vi "Test Asic Max P Min N Max N Min P.vi"(0 "Config Test IN":T1={"Config HW"={"VISA Rigol DP832"="Rigol_DP832", "Config Rigol DP832"=[{"Channel"=0, "V Limit"=5.5, "I Limit"=0.5, "V Out"=5.0}, {"Channel"=1, "V Limit"=5.5, "I Limit"=0.8, "V Out"=5.0}, {"Channel"=2, "V Limit"=5.5, "I Limit"=0.2, "V Out"=0.0}], "CTA Test#"="CTA013 A", "FT_Handle"=0, "Espera acceso FT"=10, "VISA Tek MDO3104"="Rigol_DP832", "VISA Key 81160A"="Rigol_DP832"}, "Config Test"=[{"Vasic"=2.8, "Global Reset"=FALSE, "Test Register?"=FALSE, "Test ADC?"=FALSE, "Test ADC"={"Repeats ADC"=100, "Max Desviation"=0.1}, "Limits ADC"={"Low"=[1.9, 1.3, 0.65, 0.0, 1.6, 1.4, 1.4, 0.9, 2.1, 0.85, 1.9], "High"=[2.1, 1.5, 0.85, 0.1, 1.4, 1.2, 1.2, 0.7, 1.9, 0.65, 1.7]}, "Test Max PN Min NP?"=FALSE, "Limits Max PN Min NP"={"Max P Upper"=2.177000045776367, "Min P Upper"=1.474, "Max N Upper"=1.475, "Min N Upper"=0.818, "Max P Lower"=1.888, "Min P Lower "=1.321, "Max N Lower"=1.322, "Min N Lower"=0.73}, "Test Rate Scan?"=FALSE, "Vin Rate Scan"=[], "Limits Rate Scan"={"High"=[0.15, 0.242, 0.331, 0.425, 0.512, 0.6, 0.688, 0.774, 0.847, 0.91], "Low"=[0.021, 0.11, 0.189, 0.27, 0.347, 0.421, 0.487, 0.551, 0.601, 0.635]}, "Test Rate Scan Adders?"=FALSE, "Vin Rate Adders"=[], "Limits Rate Scan adders"={"High"=[], "Low"=[]}, "Test offset analog?"=FALSE, "Lim Offset Analog"={"Max Analog"=0.05, "Min Analog"=-0.05}, "Test offset digital?"=FALSE, "Lim offset Dig"={"Max Dig"=0.05}, "Vasic real f.a."=2.8, "IBIAS"=FALSE, "VALUE IBIAS"=63}, {"Vasic"=2.8, "Global Reset"=FALSE, "Test Register?"=FALSE, "Test ADC?"=FALSE, "Test ADC"={"Repeats ADC"=100, "Max Desviation"=0.1}, "Limits ADC"={"Low"=[1.9, 1.3, 0.65, 0.0, 1.6, 1.4, 1.4, 0.9, 2.1, 0.85, 1.9], "High"=[2.1, 1.5, 0.85, 0.1, 1.4, 1.2, 1.2, 0.7, 1.9, 0.65, 1.7]}, "Test Max PN Min NP?"=FALSE, "Limits Max PN Min NP"={"Max P Upper"=2.177000045776367, "Min P Upper"=1.474, "Max N Upper"=1.475, "Min N Upper"=0.818, "Max P Lower"=1.888, "Min P Lower "=1.321, "Max N Lower"=1.322, "Min N Lower"=0.73}, "Test Rate Scan?"=FALSE, "Vin Rate Scan"=[], "Limits Rate Scan"={"High"=[0.15, 0.242, 0.331, 0.425, 0.512, 0.6, 0.688, 0.774, 0.847, 0.91], "Low"=[0.021, 0.11, 0.189, 0.27, 0.347, 0.421, 0.487, 0.551, 0.601, 0.635]}, "Test Rate Scan Adders?"=FALSE, "Vin Rate Adders"=[], "Limits Rate Scan adders"={"High"=[], "Low"=[]}, "Test offset analog?"=FALSE, "Lim Offset Analog"={"Max Analog"=0.05, "Min Analog"=-0.05}, "Test offset digital?"=FALSE, "Lim offset Dig"={"Max Dig"=0.05}, "Vasic real f.a."=2.8, "IBIAS"=FALSE, "VALUE IBIAS"=63}, {"Vasic"=2.8, "Global Reset"=FALSE, "Test Register?"=FALSE, "Test ADC?"=FALSE, "Test ADC"={"Repeats ADC"=100, "Max Desviation"=0.1}, "Limits ADC"={"Low"=[1.9, 1.3, 0.65, 0.0, 1.6, 1.4, 1.4, 0.9, 2.1, 0.85, 1.9], "High"=[2.1, 1.5, 0.85, 0.1, 1.4, 1.2, 1.2, 0.7, 1.9, 0.65, 1.7]}, "Test Max PN Min NP?"=FALSE, "Limits Max PN Min NP"={"Max P Upper"=2.177000045776367, "Min P Upper"=1.474, "Max N Upper"=1.475, "Min N Upper"=0.818, "Max P Lower"=1.888, "Min P Lower "=1.321, "Max N Lower"=1.322, "Min N Lower"=0.73}, "Test Rate Scan?"=FALSE, "Vin Rate Scan"=[], "Limits Rate Scan"={"High"=[0.15, 0.242, 0.331, 0.425, 0.512, 0.6, 0.688, 0.774, 0.847, 0.91], "Low"=[0.021, 0.11, 0.189, 0.27, 0.347, 0.421, 0.487, 0.551, 0.601, 0.635]}, "Test Rate Scan Adders?"=FALSE, "Vin Rate Adders"=[], "Limits Rate Scan adders"={"High"=[], "Low"=[]}, "Test offset analog?"=FALSE, "Lim Offset Analog"={"Max Analog"=0.05, "Min Analog"=-0.05}, "Test offset digital?"=FALSE, "Lim offset Dig"={"Max Dig"=0.05}, "Vasic real f.a."=2.8, "IBIAS"=FALSE, "VALUE IBIAS"=63}, {"Vasic"=2.8, "Global Reset"=FALSE, "Test Register?"=FALSE, "Test ADC?"=FALSE, "Test ADC"={"Repeats ADC"=100, "Max Desviation"=0.1}, "Limits ADC"={"Low"=[1.9, 1.3, 0.65, 0.0, 1.6, 1.4, 1.4, 0.9, 2.1, 0.85, 1.9], "High"=[2.1, 1.5, 0.85, 0.1, 1.4, 1.2, 1.2, 0.7, 1.9, 0.65, 1.7]}, "Test Max PN Min NP?"=FALSE, "Limits Max PN Min NP"={"Max P Upper"=2.177000045776367, "Min P Upper"=1.474, "Max N Upper"=1.475, "Min N Upper"=0.818, "Max P Lower"=1.888, "Min P Lower "=1.321, "Max N Lower"=1.322, "Min N Lower"=0.73}, "Test Rate Scan?"=FALSE, "Vin Rate Scan"=[], "Limits Rate Scan"={"High"=[0.15, 0.242, 0.331, 0.425, 0.512, 0.6, 0.688, 0.774, 0.847, 0.91], "Low"=[0.021, 0.11, 0.189, 0.27, 0.347, 0.421, 0.487, 0.551, 0.601, 0.635]}, "Test Rate Scan Adders?"=FALSE, "Vin Rate Adders"=[], "Limits Rate Scan adders"={"High"=[], "Low"=[]}, "Test offset analog?"=FALSE, "Lim Offset Analog"={"Max Analog"=0.05, "Min Analog"=-0.05}, "Test offset digital?"=FALSE, "Lim offset Dig"={"Max Dig"=0.05}, "Vasic real f.a."=2.8, "IBIAS"=FALSE, "VALUE IBIAS"=63}], "Result"=[], "Execucion Test"={"Vasic Actual"=0}, "Config VGA"={"Theoretical Voltage"=[], "Real Voltage"=[102.85, 207.14, 299.57, 404.85, 495.71, 606.85, 697.71, 801.14, 897.14, 998.85], "Pulse Width"=57344, "Frecuency Pulse"=1000000.0, "VGA Gain"=[9, 16, 24, 34, 43, 52, 61, 72, 81, 93]}, "Test Info"={"Asic"="", "Operator"="", "Place"="", "Time start"=timestamp(0 s since 1904-01-01), "Time stop"=timestamp(0 s since 1904-01-01)}, "Info machine"={"SO"="", "SO Name"="", "SO Ver"="", "SO Build"="", "CPU"="", "APP"="", "APP YEAR"="", "APP ver"="", "APP User"="", "APP Serail"="", "MAC"=[], "PC NAME"=[], "PC IP"=[], "BIOS MANU"="", "BIOS NAME"="", "BIOS SERIAL"="", "BOARD MANU"="", "BOARD NAME"="", "BOARD SERIAL"="", "Driver Version"="", "Library Version"="", "FPGA Ver"=0, "ID CTA board"=0, "LAST BOOT"="", "LABVIEW Ver"=0}, "Partial Report"="", "CONFIG GEN"=[]} {"CONFIG GEN"."Vasic Theorical" min=1.0 max=1000000.0 step=1.0 format="%#_6pV"; "CONFIG GEN"."Frequency" min=0.001 max=333000000.0 step=1000.0 format="%#_6pHz"; "CONFIG GEN"."Leading Edge Time" min=1e-09 max=1.0 step=1e-10 format="%#_6ps"; "CONFIG GEN"."Trailing Edge Time" min=1e-09 max=1.0 step=1e-10 format="%#_6ps"; "CONFIG GEN"."Delay" min=0.0 max=1.0 step=1e-12 format="%#_6ps"; "CONFIG GEN"."Trigger Level Sync" items=["ECL", "TTL"]; "CONFIG GEN"."Trigger Sync Out" items=["AB"=3, "B"=2, "A"=1, "None"=0]; "CONFIG GEN"."Load" min=1.0 max=1000000.0 step=1.0 format="%#_6p"; "CONFIG GEN"."DC Offset" min=-10.0 max=10.0 step=0.1 format="%#_6pV"; "CONFIG GEN"."Amplitude" min=0.05 max=5.0 step=0.001 format="%#_6pV"; "CONFIG GEN"."Width Time" min=1.5e-09 max=1.0 step=1e-10 format="%#_6ps"; "CONFIG GEN"."Channel" items=["Channel1"=1, "Channel2"=2]; "Config VGA"."Theoretical Voltage" format="%1.4f"; "Config VGA"."VGA Gain" format="%02x"; "Config VGA"."Frecuency Pulse" format="%0_2p"; "Config VGA"."Pulse Width" format="%04x"; "Config VGA"."Real Voltage" format="%1.5f"; "Config Test"."VALUE IBIAS" max=63 step=1; "Config Test"."Vasic real f.a." min=2.8 max=3.8 step=0.01 format="%.2g"; "Config Test"."Limits Rate Scan adders"."Low" format="%1.3f"; "Config Test"."Limits Rate Scan adders"."High" format="%1.3f"; "Config Test"."Limits ADC"."High" format="%1.4f"; "Config Test"."Limits ADC"."Low" format="%1.3f"; "Config Test"."Lim offset Dig"."Max Dig" format="%.3g"; "Config Test"."Lim Offset Analog"."Min Analog" format="%.3g"; "Config Test"."Lim Offset Analog"."Max Analog" format="%.3g"; "Config Test"."Limits Rate Scan"."Low" format="%1.4f"; "Config Test"."Limits Rate Scan"."High" format="%1.3f"; "Config Test"."Limits Max PN Min NP"."Min P Upper" format="%.3g"; "Config Test"."Limits Max PN Min NP"."Min P Lower" format="%.3g"; "Config Test"."Limits Max PN Min NP"."Max N Lower" format="%.3g"; "Config Test"."Limits Max PN Min NP"."Max N Upper" format="%.3g"; "Config Test"."Limits Max PN Min NP"."Min N Lower" format="%.3g"; "Config Test"."Limits Max PN Min NP"."Min N Upper" format="%.3g"; "Config Test"."Limits Max PN Min NP"."Max P Upper" format="%.3g"; "Config Test"."Limits Max PN Min NP"."Max P Lower" format="%.3g"; "Config Test"."Vasic" min=2.8 max=3.8 step=0.01 format="%.2g"; "Config HW"."Config Rigol DP832"."Channel" items=["+30V Channel 1", "+30V Channel 2", "+5V Channel 3"]; "Config HW"."Config Rigol DP832"."V Limit" format="%.1g"; "Config HW"."Config Rigol DP832"."I Limit" format="%.1g"; "Config HW"."Config Rigol DP832"."V Out" format="%.1g"; "Result"."Test Registros"."Read W/R" format="%04x"; "Result"."Test Registros"."Pattern W/R" format="%04x"; "Result"."Test Registros"."Read Default" format="%04x"; "Result"."Test Registros"."Pattern Default" format="%04x"}, 11 "Error IN":errorcluster) -> (4 "Config Test OUT":T1={"Config HW"={"VISA Rigol DP832"="Rigol_DP832", "Config Rigol DP832"=[{"Channel"=0, "V Limit"=5.5, "I Limit"=0.5, "V Out"=5.0}, {"Channel"=1, "V Limit"=5.5, "I Limit"=0.8, "V Out"=5.0}, {"Channel"=2, "V Limit"=5.5, "I Limit"=0.2, "V Out"=0.0}], "CTA Test#"="CTA013 A", "FT_Handle"=0, "Espera acceso FT"=10, "VISA Tek MDO3104"="Rigol_DP832", "VISA Key 81160A"="Rigol_DP832"}, "Config Test"=[{"Vasic"=2.8, "Global Reset"=FALSE, "Test Register?"=FALSE, "Test ADC?"=FALSE, "Test ADC"={"Repeats ADC"=100, "Max Desviation"=0.1}, "Limits ADC"={"Low"=[1.9, 1.3, 0.65, 0.0, 1.6, 1.4, 1.4, 0.9, 2.1, 0.85, 1.9], "High"=[2.1, 1.5, 0.85, 0.1, 1.4, 1.2, 1.2, 0.7, 1.9, 0.65, 1.7]}, "Test Max PN Min NP?"=FALSE, "Limits Max PN Min NP"={"Max P Upper"=2.177000045776367, "Min P Upper"=1.474, "Max N Upper"=1.475, "Min N Upper"=0.818, "Max P Lower"=1.888, "Min P Lower "=1.321, "Max N Lower"=1.322, "Min N Lower"=0.73}, "Test Rate Scan?"=FALSE, "Vin Rate Scan"=[], "Limits Rate Scan"={"High"=[0.15, 0.242, 0.331, 0.425, 0.512, 0.6, 0.688, 0.774, 0.847, 0.91], "Low"=[0.021, 0.11, 0.189, 0.27, 0.347, 0.421, 0.487, 0.551, 0.601, 0.635]}, "Test Rate Scan Adders?"=FALSE, "Vin Rate Adders"=[], "Limits Rate Scan adders"={"High"=[], "Low"=[]}, "Test offset analog?"=FALSE, "Lim Offset Analog"={"Max Analog"=0.05, "Min Analog"=-0.05}, "Test offset digital?"=FALSE, "Lim offset Dig"={"Max Dig"=0.05}, "Vasic real f.a."=2.8, "IBIAS"=FALSE, "VALUE IBIAS"=63}, {"Vasic"=2.8, "Global Reset"=FALSE, "Test Register?"=FALSE, "Test ADC?"=FALSE, "Test ADC"={"Repeats ADC"=100, "Max Desviation"=0.1}, "Limits ADC"={"Low"=[1.9, 1.3, 0.65, 0.0, 1.6, 1.4, 1.4, 0.9, 2.1, 0.85, 1.9], "High"=[2.1, 1.5, 0.85, 0.1, 1.4, 1.2, 1.2, 0.7, 1.9, 0.65, 1.7]}, "Test Max PN Min NP?"=FALSE, "Limits Max PN Min NP"={"Max P Upper"=2.177000045776367, "Min P Upper"=1.474, "Max N Upper"=1.475, "Min N Upper"=0.818, "Max P Lower"=1.888, "Min P Lower "=1.321, "Max N Lower"=1.322, "Min N Lower"=0.73}, "Test Rate Scan?"=FALSE, "Vin Rate Scan"=[], "Limits Rate Scan"={"High"=[0.15, 0.242, 0.331, 0.425, 0.512, 0.6, 0.688, 0.774, 0.847, 0.91], "Low"=[0.021, 0.11, 0.189, 0.27, 0.347, 0.421, 0.487, 0.551, 0.601, 0.635]}, "Test Rate Scan Adders?"=FALSE, "Vin Rate Adders"=[], "Limits Rate Scan adders"={"High"=[], "Low"=[]}, "Test offset analog?"=FALSE, "Lim Offset Analog"={"Max Analog"=0.05, "Min Analog"=-0.05}, "Test offset digital?"=FALSE, "Lim offset Dig"={"Max Dig"=0.05}, "Vasic real f.a."=2.8, "IBIAS"=FALSE, "VALUE IBIAS"=63}, {"Vasic"=2.8, "Global Reset"=FALSE, "Test Register?"=FALSE, "Test ADC?"=FALSE, "Test ADC"={"Repeats ADC"=100, "Max Desviation"=0.1}, "Limits ADC"={"Low"=[1.9, 1.3, 0.65, 0.0, 1.6, 1.4, 1.4, 0.9, 2.1, 0.85, 1.9], "High"=[2.1, 1.5, 0.85, 0.1, 1.4, 1.2, 1.2, 0.7, 1.9, 0.65, 1.7]}, "Test Max PN Min NP?"=FALSE, "Limits Max PN Min NP"={"Max P Upper"=2.177000045776367, "Min P Upper"=1.474, "Max N Upper"=1.475, "Min N Upper"=0.818, "Max P Lower"=1.888, "Min P Lower "=1.321, "Max N Lower"=1.322, "Min N Lower"=0.73}, "Test Rate Scan?"=FALSE, "Vin Rate Scan"=[], "Limits Rate Scan"={"High"=[0.15, 0.242, 0.331, 0.425, 0.512, 0.6, 0.688, 0.774, 0.847, 0.91], "Low"=[0.021, 0.11, 0.189, 0.27, 0.347, 0.421, 0.487, 0.551, 0.601, 0.635]}, "Test Rate Scan Adders?"=FALSE, "Vin Rate Adders"=[], "Limits Rate Scan adders"={"High"=[], "Low"=[]}, "Test offset analog?"=FALSE, "Lim Offset Analog"={"Max Analog"=0.05, "Min Analog"=-0.05}, "Test offset digital?"=FALSE, "Lim offset Dig"={"Max Dig"=0.05}, "Vasic real f.a."=2.8, "IBIAS"=FALSE, "VALUE IBIAS"=63}, {"Vasic"=2.8, "Global Reset"=FALSE, "Test Register?"=FALSE, "Test ADC?"=FALSE, "Test ADC"={"Repeats ADC"=100, "Max Desviation"=0.1}, "Limits ADC"={"Low"=[1.9, 1.3, 0.65, 0.0, 1.6, 1.4, 1.4, 0.9, 2.1, 0.85, 1.9], "High"=[2.1, 1.5, 0.85, 0.1, 1.4, 1.2, 1.2, 0.7, 1.9, 0.65, 1.7]}, "Test Max PN Min NP?"=FALSE, "Limits Max PN Min NP"={"Max P Upper"=2.177000045776367, "Min P Upper"=1.474, "Max N Upper"=1.475, "Min N Upper"=0.818, "Max P Lower"=1.888, "Min P Lower "=1.321, "Max N Lower"=1.322, "Min N Lower"=0.73}, "Test Rate Scan?"=FALSE, "Vin Rate Scan"=[], "Limits Rate Scan"={"High"=[0.15, 0.242, 0.331, 0.425, 0.512, 0.6, 0.688, 0.774, 0.847, 0.91], "Low"=[0.021, 0.11, 0.189, 0.27, 0.347, 0.421, 0.487, 0.551, 0.601, 0.635]}, "Test Rate Scan Adders?"=FALSE, "Vin Rate Adders"=[], "Limits Rate Scan adders"={"High"=[], "Low"=[]}, "Test offset analog?"=FALSE, "Lim Offset Analog"={"Max Analog"=0.05, "Min Analog"=-0.05}, "Test offset digital?"=FALSE, "Lim offset Dig"={"Max Dig"=0.05}, "Vasic real f.a."=2.8, "IBIAS"=FALSE, "VALUE IBIAS"=63}], "Result"=[], "Execucion Test"={"Vasic Actual"=0}, "Config VGA"={"Theoretical Voltage"=[], "Real Voltage"=[102.85, 207.14, 299.57, 404.85, 495.71, 606.85, 697.71, 801.14, 897.14, 998.85], "Pulse Width"=57344, "Frecuency Pulse"=1000000.0, "VGA Gain"=[9, 16, 24, 34, 43, 52, 61, 72, 81, 93]}, "Test Info"={"Asic"="", "Operator"="", "Place"="", "Time start"=timestamp(0 s since 1904-01-01), "Time stop"=timestamp(0 s since 1904-01-01)}, "Info machine"={"SO"="", "SO Name"="", "SO Ver"="", "SO Build"="", "CPU"="", "APP"="", "APP YEAR"="", "APP ver"="", "APP User"="", "APP Serail"="", "MAC"=[], "PC NAME"=[], "PC IP"=[], "BIOS MANU"="", "BIOS NAME"="", "BIOS SERIAL"="", "BOARD MANU"="", "BOARD NAME"="", "BOARD SERIAL"="", "Driver Version"="", "Library Version"="", "FPGA Ver"=0, "ID CTA board"=0, "LAST BOOT"="", "LABVIEW Ver"=0}, "Partial Report"="", "CONFIG GEN"=[]} {"CONFIG GEN"."Vasic Theorical" min=1.0 max=1000000.0 step=1.0 format="%#_6pV"; "CONFIG GEN"."Frequency" min=0.001 max=333000000.0 step=1000.0 format="%#_6pHz"; "CONFIG GEN"."Leading Edge Time" min=1e-09 max=1.0 step=1e-10 format="%#_6ps"; "CONFIG GEN"."Trailing Edge Time" min=1e-09 max=1.0 step=1e-10 format="%#_6ps"; "CONFIG GEN"."Delay" min=0.0 max=1.0 step=1e-12 format="%#_6ps"; "CONFIG GEN"."Trigger Level Sync" items=["ECL", "TTL"]; "CONFIG GEN"."Trigger Sync Out" items=["AB"=3, "B"=2, "A"=1, "None"=0]; "CONFIG GEN"."Load" min=1.0 max=1000000.0 step=1.0 format="%#_6p"; "CONFIG GEN"."DC Offset" min=-10.0 max=10.0 step=0.1 format="%#_6pV"; "CONFIG GEN"."Amplitude" min=0.05 max=5.0 step=0.001 format="%#_6pV"; "CONFIG GEN"."Width Time" min=1.5e-09 max=1.0 step=1e-10 format="%#_6ps"; "CONFIG GEN"."Channel" items=["Channel1"=1, "Channel2"=2]; "Config VGA"."Theoretical Voltage" format="%1.4f"; "Config VGA"."VGA Gain" format="%02x"; "Config VGA"."Frecuency Pulse" format="%0_2p"; "Config VGA"."Pulse Width" format="%04x"; "Config VGA"."Real Voltage" format="%1.5f"; "Config Test"."VALUE IBIAS" max=63 step=1; "Config Test"."Vasic real f.a." min=2.8 max=3.8 step=0.01 format="%.2g"; "Config Test"."Limits Rate Scan adders"."Low" format="%1.3f"; "Config Test"."Limits Rate Scan adders"."High" format="%1.3f"; "Config Test"."Limits ADC"."High" format="%1.4f"; "Config Test"."Limits ADC"."Low" format="%1.3f"; "Config Test"."Lim offset Dig"."Max Dig" format="%.3g"; "Config Test"."Lim Offset Analog"."Min Analog" format="%.3g"; "Config Test"."Lim Offset Analog"."Max Analog" format="%.3g"; "Config Test"."Limits Rate Scan"."Low" format="%1.4f"; "Config Test"."Limits Rate Scan"."High" format="%1.3f"; "Config Test"."Limits Max PN Min NP"."Min P Upper" format="%.3g"; "Config Test"."Limits Max PN Min NP"."Min P Lower" format="%.3g"; "Config Test"."Limits Max PN Min NP"."Max N Lower" format="%.3g"; "Config Test"."Limits Max PN Min NP"."Max N Upper" format="%.3g"; "Config Test"."Limits Max PN Min NP"."Min N Lower" format="%.3g"; "Config Test"."Limits Max PN Min NP"."Min N Upper" format="%.3g"; "Config Test"."Limits Max PN Min NP"."Max P Upper" format="%.3g"; "Config Test"."Limits Max PN Min NP"."Max P Lower" format="%.3g"; "Config Test"."Vasic" min=2.8 max=3.8 step=0.01 format="%.2g"; "Config HW"."Config Rigol DP832"."Channel" items=["+30V Channel 1", "+30V Channel 2", "+5V Channel 3"]; "Config HW"."Config Rigol DP832"."V Limit" format="%.1g"; "Config HW"."Config Rigol DP832"."I Limit" format="%.1g"; "Config HW"."Config Rigol DP832"."V Out" format="%.1g"; "Result"."Test Registros"."Read W/R" format="%04x"; "Result"."Test Registros"."Pattern W/R" format="%04x"; "Result"."Test Registros"."Read Default" format="%04x"; "Result"."Test Registros"."Pattern Default" format="%04x"}, 8 "Max P Min N":bool, 10 "Min P Max N":bool, 15 "Error OUT":errorcluster)   [LabVIEW 2019]
uses:
  Test.ctl
  TEST.TEST CONFIG HW.ctl
  Rigol DP832/DP832_Control Channels.ctl
  TEST.TEST CONFIG TEST MATRIZ.ctl
  TEST.TEST CONFIG TEST.ctl
  TEST.TEST RESULT.ctl
  test_result fvasic.ctl
  TEST.TEST EXECUTION TEST.ctl
  TEST.TEST CONFIG VGA.ctl
  TEST.TEST TEST INFO.ctl
  TEST.TEST INFO PC.ctl
  GenPulse_configurar.ctl
  Global.Salir Ya.vi
panel:
  in  "Tab Control":enum32{"Page 1", "Page 2"}(tab)
  out "Progress %":u8 format="%02d%%"
  out "Progress barr":u8(slide) scale=0.0..100.0
  # "Test Max P Min N / Min P Max N"
  # "Modo 2\nModo 3\nModo 4\nModo 2\nModo 3\nModo 4"
  # "Modo 2\nModo 3\nModo 4\nModo 2\nModo 3\nModo 4"
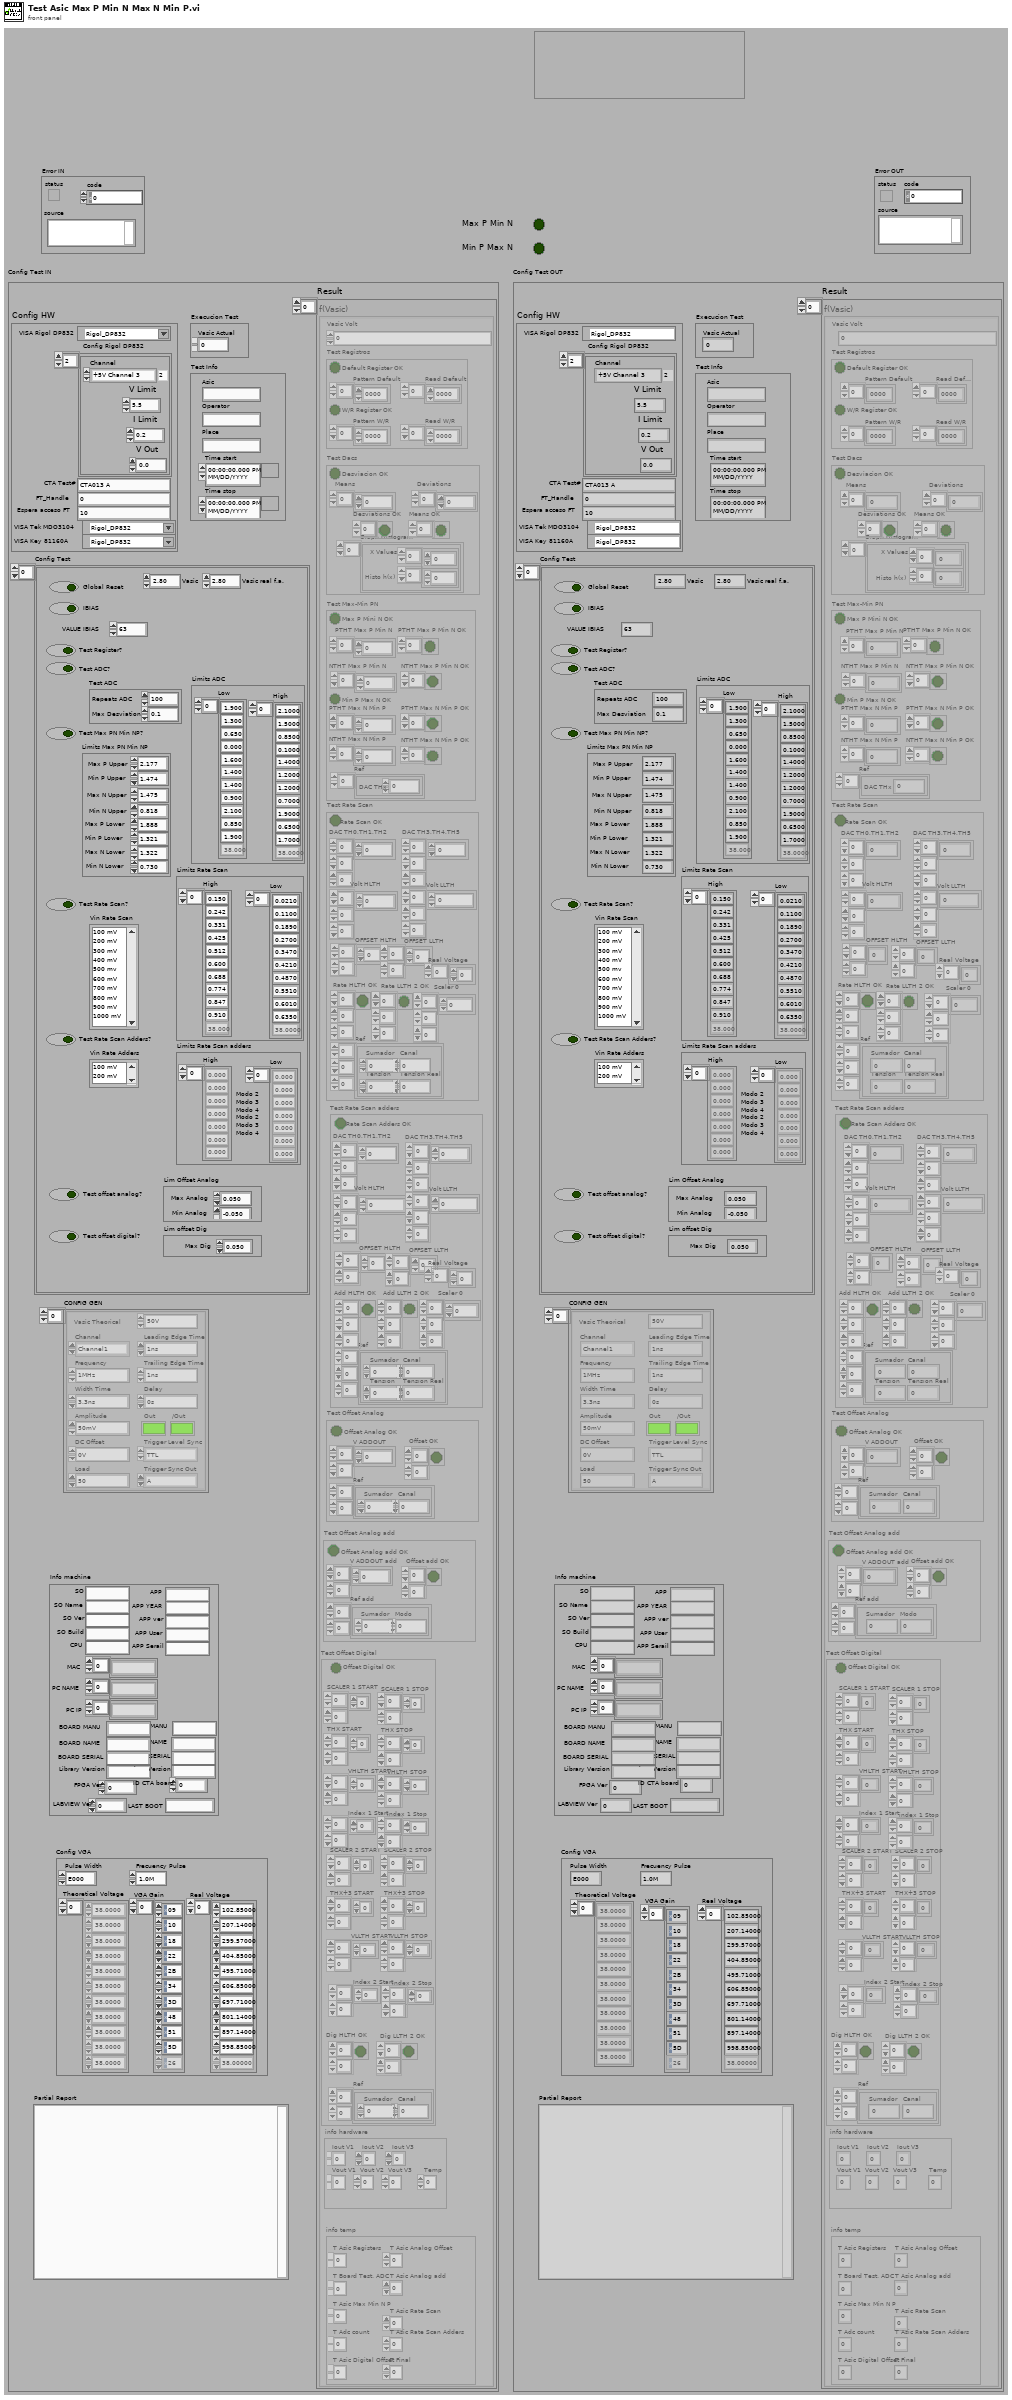
[diagram p1: front panel]
types:
  T1 = typedef "Test.ctl" = cluster{"Config HW":T2, "Config Test":T4, "Result":T6, "Execucion Test":T8, "Config VGA":T9, "Test Info":T10, "Info machine":T11, "Partial Report":string, "CONFIG GEN":T12[]}
  T2 = typedef "TEST.TEST CONFIG HW.ctl" = cluster{"VISA Rigol DP832":refnum<visa-resource-name>, "Config Rigol DP832":cluster{"Channel":T3, "V Limit":dbl, "I Limit":dbl, "V Out":dbl}[], "CTA Test#":string, "FT_Handle":u32, "Espera acceso FT":u32, "VISA Tek MDO3104":refnum<visa-resource-name>, "VISA Key 81160A":refnum<visa-resource-name>}
  T3 = typedef "DP832_Control Channels.ctl" = i32
  T4 = typedef "TEST.TEST CONFIG TEST MATRIZ.ctl" = T5[]
  T5 = typedef "TEST.TEST CONFIG TEST.ctl" = cluster{"Vasic":dbl, "Global Reset":bool, "Test Register?":bool, "Test ADC?":bool, "Test ADC":cluster{"Repeats ADC":i32, "Max Desviation":dbl}, "Limits ADC":cluster{"Low":dbl[], "High":dbl[]}, "Test Max PN Min NP?":bool, "Limits Max PN Min NP":cluster{"Max P Upper":dbl, "Min P Upper":dbl, "Max N Upper":dbl, "Min N Upper":dbl, "Max P Lower":dbl, "Min P Lower ":dbl, "Max N Lower":dbl, "Min N Lower":dbl}, "Test Rate Scan?":bool, "Vin Rate Scan":i32[], "Limits Rate Scan":cluster{"High":dbl[], "Low":dbl[]}, "Test Rate Scan Adders?":bool, "Vin Rate Adders":i32[], "Limits Rate Scan adders":cluster{"High":dbl[], "Low":dbl[]}, "Test offset analog?":bool, "Lim Offset Analog":cluster{"Max Analog":dbl, "Min Analog":dbl}, "Test offset digital?":bool, "Lim offset Dig":cluster{"Max Dig":dbl}, "Vasic real f.a.":dbl, "IBIAS":bool, "VALUE IBIAS":u8}
  T6 = typedef "TEST.TEST RESULT.ctl" = T7[]
  T7 = typedef "test_result fvasic.ctl" = cluster{"Vasic Volt":i32, "Test Registros":cluster{"Default Register OK":bool, "Pattern Default":u16[], "Read Default":u16[], "W/R Register OK":bool, "Pattern W/R":u16[], "Read W/R":u16[]}, "Test Dacs":cluster{"Desviacion OK":bool, "Means":dbl[], "Deviations":dbl[], "Desviations OK":bool[], "Means OK":bool[], "Graph Histogram":cluster{"X Values":dbl[], "Histo h(x)":i32[]}[]}, "Test Max-Min PN":cluster{"Max P Mini N OK":bool, "PTHT Max P Min N":dbl[], "PTHT Max P Min N OK":bool[], "NTHT Max P Min N":dbl[], "NTHT Max P Min N OK":bool[], "Min P Max N OK":bool, "PTHT Max N Min P":dbl[], "PTHT Max N Min P OK":bool[], "NTHT Max N Min P":dbl[], "NTHT Max N Min P OK":bool[], "Ref":cluster{"DAC THx":u8}[]}, "Test Rate Scan":cluster{"Rate Scan OK":bool, "DAC TH0,TH1,TH2":u16[][][], "Volt HLTH":dbl[][][], "Rate HLTH OK":bool[][][], "DAC TH3,TH4,TH5":u16[][][], "Volt LLTH":dbl[][][], "Rate LLTH 2 OK":bool[][][], "Scaler 0":u16[][][], "Ref":cluster{"Sumador":u8, "Canal":u8, "Tension":u8, "Tension Real":dbl}[][][], "OFFSET HLTH":dbl[][], "OFFSET LLTH":dbl[][], "Real Voltage":dbl[]}, "Test Rate Scan adders":cluster{"Rate Scan Adders OK":bool, "DAC TH0,TH1,TH2":u16[][][], "Volt HLTH":dbl[][][], "Add HLTH OK":bool[][][], "DAC TH3,TH4,TH5":u16[][][], "Volt LLTH":dbl[][][], "Add LLTH 2 OK":bool[][][], "Scaler 0":u16[][][], "Ref":cluster{"Sumador":u8, "Canal":u8, "Tension":u8, "Tension Real":dbl}[][][], "OFFSET HLTH":dbl[][], "OFFSET LLTH":dbl[][], "Real Voltage":dbl[]}, "Test Offset Analog":cluster{"Offset Analog OK":bool, "V ADDOUT":dbl[][], "Offset OK":bool[][], "Ref":cluster{"Sumador":u8, "Canal":u8}[][]}, "Test Offset Digital":cluster{"Offset Digital OK":bool, "SCALER 1 START":u16[][], "SCALER 1 STOP":u16[][], "THX START":u16[][], "THX STOP":u16[][], "VHLTH START":dbl[][], "VHLTH STOP":dbl[][], "Index 1 Start":i32[][], "index 1 Stop":i32[][], "SCALER 2 START":u16[][], "SCALER 2 STOP":u16[][], "THX+3 START":u16[][], "THX+3 STOP":u16[][], "VLLTH START":dbl[][], "VLLTH STOP":dbl[][], "Index 2 Start":i32[][], "index 2 Stop":i32[][], "Dig HLTH OK":bool[][], "Dig LLTH 2 OK":bool[][], "Ref":cluster{"Sumador":u8, "Canal":u8}[][]}, "info hardware":cluster{"Iout V1":dbl, "Iout V2":dbl, "Iout V3":dbl, "Vout V1":dbl, "Vout V2":dbl, "Vout V3":dbl, "Temp":dbl}, "Test Offset Analog add":cluster{"Offset Analog add OK":bool, "V ADDOUT add":dbl[][], "Offset add OK":bool[][], "Ref add":cluster{"Sumador":u8, "Modo":u8}[][]}, "info temp":cluster{"T Asic Registers":dbl, "T Board Test. ADC":dbl, "T Asic Max Min N P":dbl, "T Adc count":dbl, "T Asic Digital Offset":dbl, "T Asic Analog Offset":dbl, "T Asic Analog add":dbl, "T Asic Rate Scan":dbl, "T Asic Rate Scan Adders":dbl, "T Final":dbl}}
  T8 = typedef "TEST.TEST EXECUTION TEST.ctl" = cluster{"Vasic Actual":i32}
  T9 = typedef "TEST.TEST CONFIG VGA.ctl" = cluster{"Theoretical Voltage":dbl[], "Real Voltage":dbl[], "Pulse Width":u16, "Frecuency Pulse":dbl, "VGA Gain":u8[]}
  T10 = typedef "TEST.TEST TEST INFO.ctl" = cluster{"Asic":string, "Operator":string, "Place":string, "Time start":timestamp, "Time stop":timestamp}
  T11 = typedef "TEST.TEST INFO PC.ctl" = cluster{"SO":string, "SO Name":string, "SO Ver":string, "SO Build":string, "CPU":string, "APP":string, "APP YEAR":string, "APP ver":string, "APP User":string, "APP Serail":string, "MAC":string[], "PC NAME":string[], "PC IP":string[], "BIOS MANU":string, "BIOS NAME":string, "BIOS SERIAL":string, "BOARD MANU":string, "BOARD NAME":string, "BOARD SERIAL":string, "Driver Version":string, "Library Version":string, "FPGA Ver":u8, "ID CTA board":u64, "LAST BOOT":string, "LABVIEW Ver":u32}
  T12 = typedef "GenPulse_configurar.ctl" = cluster{"Channel":u16, "Frequency":dbl, "Width Time":dbl, "Amplitude":dbl, "DC Offset":dbl, "Load":dbl, "Leading Edge Time":dbl, "Trailing Edge Time":dbl, "Delay":dbl, "Out":bool, "/Out":bool, "Trigger Level Sync":u16, "Trigger Sync Out":u16, "Vasic Theorical":dbl}
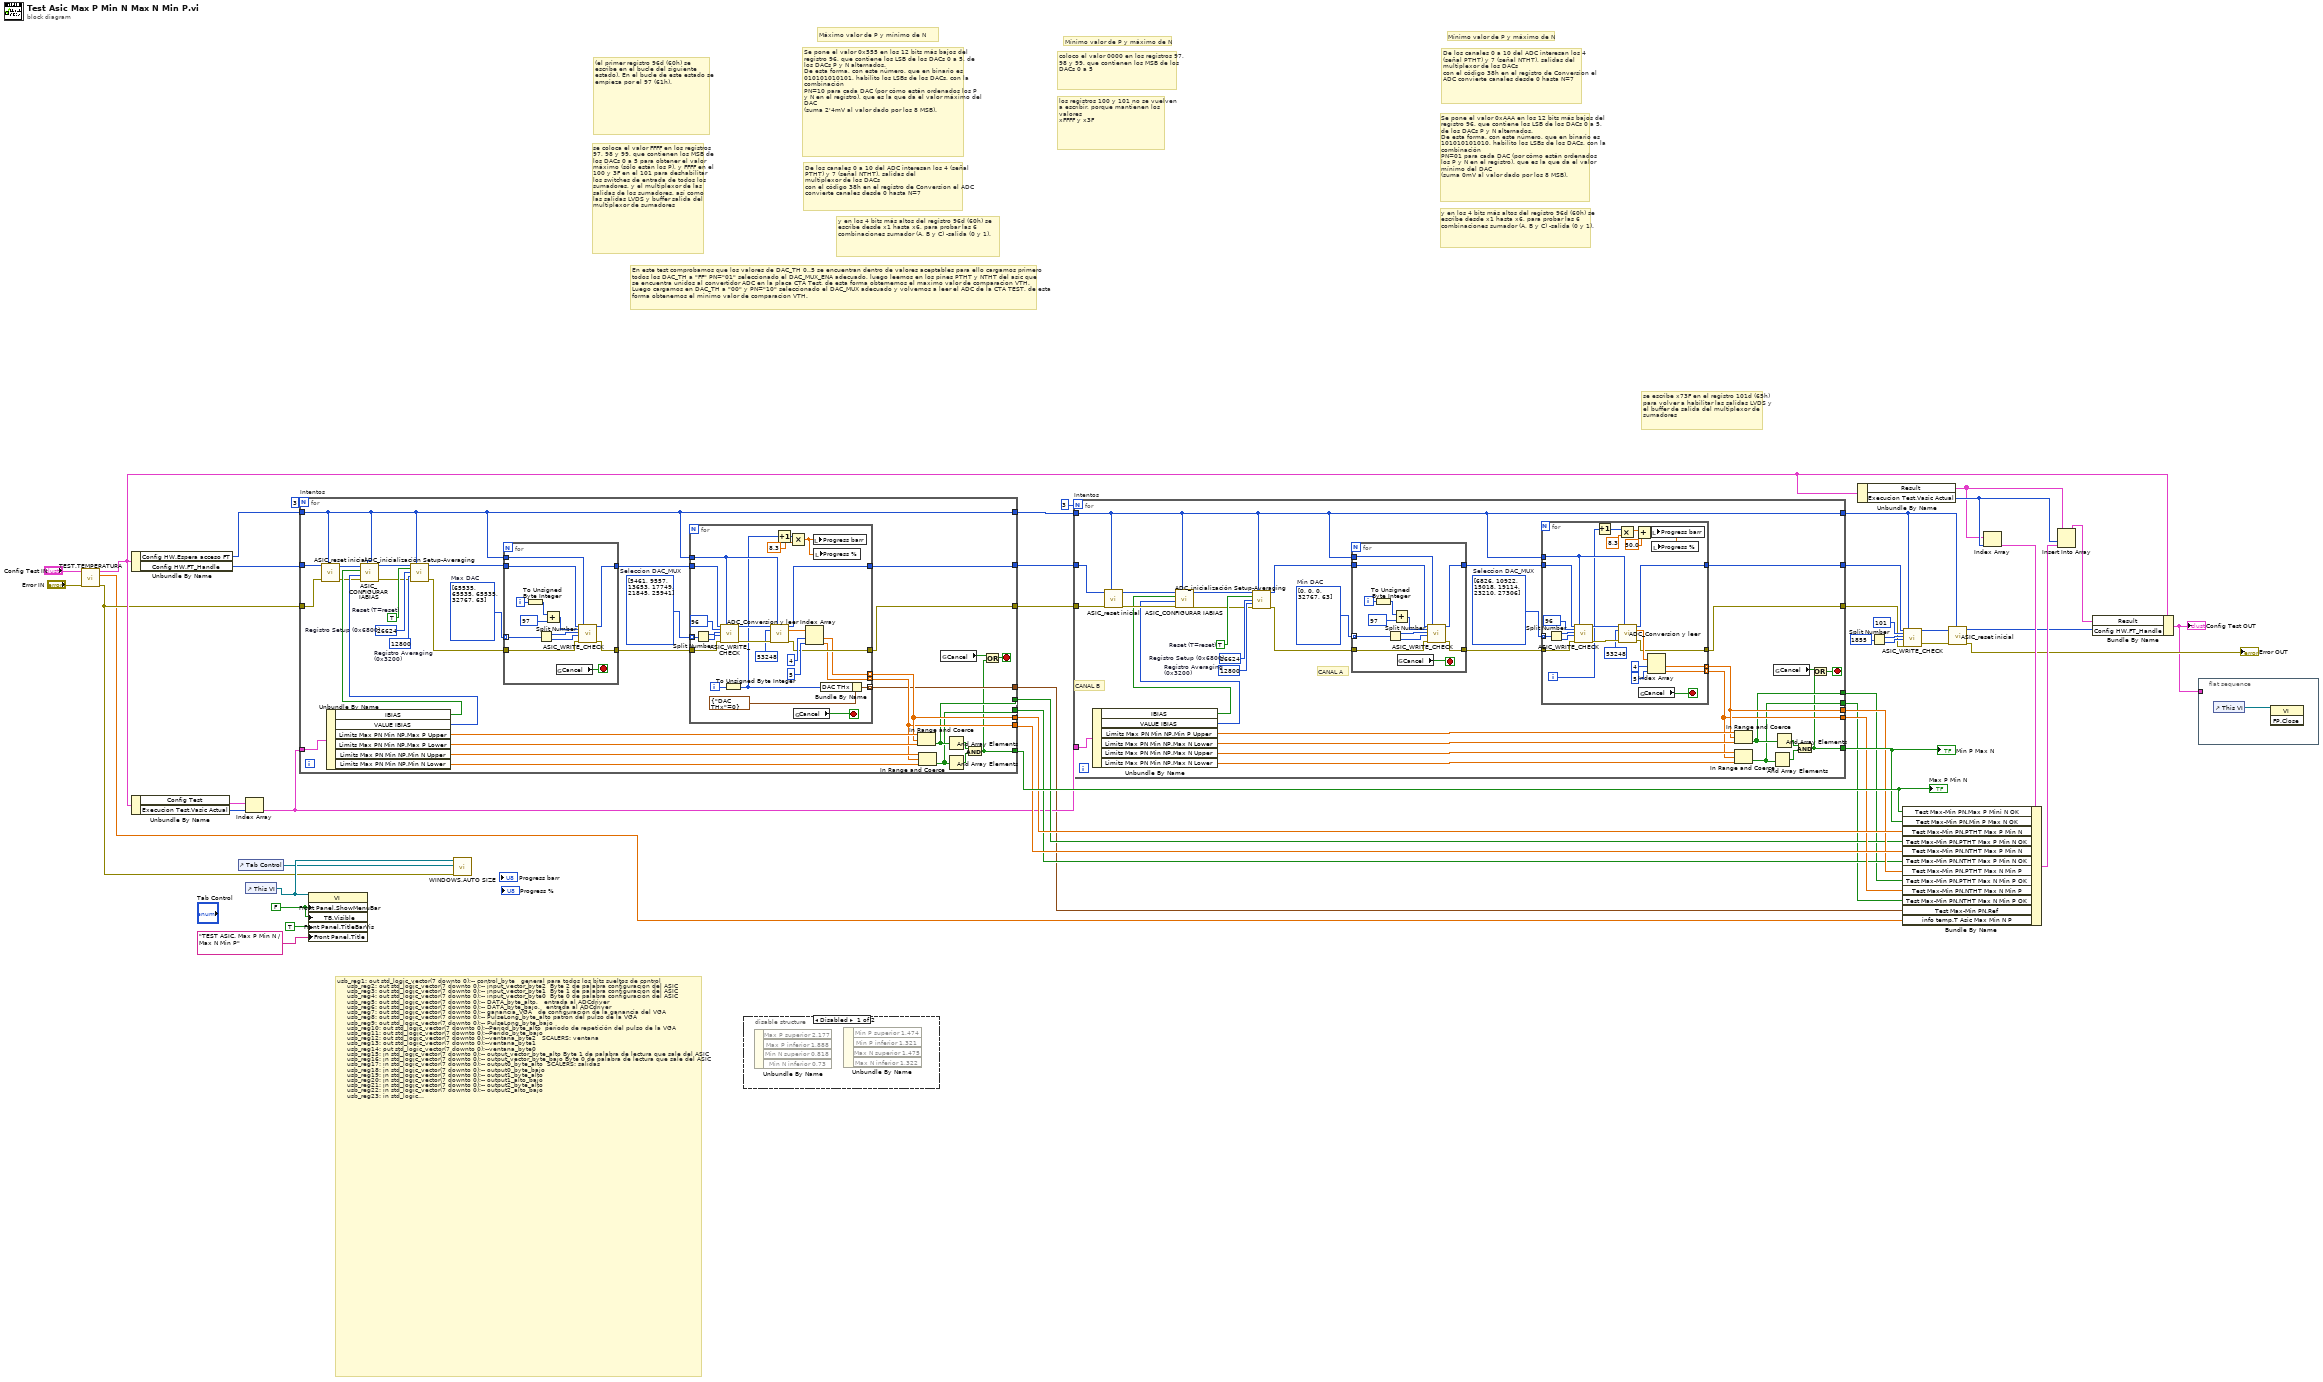
[diagram p0: block diagram]
diagram:
  w23 = FALSE ("Front Panel Window:Show Menu Bar")
  # "En este test comprobamos que los valores de DAC_TH 0..5 se encuentran dentro de valores aceptables para ello cargamos primero\ntodos los DAC_TH a \"FF\" PN=\"01\" seleccionado el DAC_MUX_ENA adecuado, luego leemos en los pines PTHT y NTHT del asic que \nse encuentra unidos al convertidor ADC en la placa CTA Test, de esta forma obtememos el maximo valor de comparacion VTH.\nLuego cargamos en DAC_TH a \"00\" y PN=\"10\" seleccionado el DAC_MUX adecuado y volvemos a leer el ADC de la CTA TEST, de esta\nforma obtenemos el minimo valor de comparacion VTH."
  # "se escribe x73F en el registro 101d (65h) para volver a habilitar las salidas LVDS y el buffer de salida del multiplexor de sumadores"
  # "Mínimo valor de P y máximo de N"
  # "De los canales 0 a 10 del ADC interesan los 4 (señal PTHT) y 7 (señal NTHT), salidas del\nmultiplexor de los DACs\ncon el código 38h en el registro de Conversion el ADC convierte canales desde 0 hasta N=7"
  # "Se pone el valor 0xAAA en los 12 bits más bajos del registro 96, que contiene los LSB de los DACs 0 a 5, de los DACs P y N alternados.\nDe esta forma, con este número, que en binario es 101010101010, habilito los LSBs de los DACs, con la combinación\nPN=01 para cada DAC (por cómo están ordenados los P y N en el registro), que es la que da el valor mínimo del DAC \n(suma 0mV al valor dado por los 8 MSB)."
  # "y en los 4 bits más altos del registro 96d (60h) se escribe desde x1 hasta x6, para probar las 6 combinaciones sumador (A, B y C) -salida (0 y 1)."
  # "los registros 100 y 101 no se vuelven \na escribir, porque mantienen los valores \nxFFFF y x3F"
  # "coloco el valor 0000 en los registros 97, 98 y 99, que contienen los MSB de los DACs 0 a 5"
  # "Mínimo valor de P y máximo de N"
  # "y en los 4 bits más altos del registro 96d (60h) se escribe desde x1 hasta x6, para probar las 6 combinaciones sumador (A, B y C) -salida (0 y 1)."
  # "Se pone el valor 0x555 en los 12 bits más bajos del registro 96, que contiene los LSB de los DACs 0 a 5, de los DACs P y N alternados.\nDe esta forma, con este número, que en binario es 010101010101, habilito los LSBs de los DACs, con la combinación\nPN=10 para cada DAC (por cómo están ordenados los P y N en el registro), que es la que da el valor máximo del DAC \n(suma 2'4mV al valor dado por los 8 MSB)."
  # "Máximo valor de P y mínimo de N"
  # "De los canales 0 a 10 del ADC interesan los 4 (señal PTHT) y 7 (señal NTHT), salidas del\nmultiplexor de los DACs\ncon el código 38h en el registro de Conversion el ADC convierte canales desde 0 hasta N=7"
  # "(el primer registro 96d (60h) se\nescribe en el bucle del siguiente \nestado). En el bucle de este estado se empieza por el 97 (61h)."
  # "se coloca el valor FFFF en los registros 97, 98 y 99, que contienen los MSB de los DACs 0 a 5 para obtener el valor máximo (sólo están los P), y FFFF en el 100 y 3F en el 101 para deshabilitar los switches de entrada de todos los sumadores, y el multiplexor de las salidas de los sumadores, así como las salidas LVDS y buffer salida del multiplexor de sumadores"
  # "usb_reg1: out std_logic_vector(7 downto 0);-- control_byte\t\t\tgeneral para todos los bits sueltos de control\n\t\t\t  usb_reg2: out std_logic_vector(7 downto 0);-- input_vector_byte2 \tByte 2 de palabra configuración del ASIC\n\t\t\t  usb_reg3: out std_logic_vector(7 downto 0);-- input_vector_byte1 \tByte 1 de palabra configuración del ASIC\n\t\t\t  usb_reg4: out std_logic_vector(7 downto 0);-- input_vector_byte0 \tByte 0 de palabra configuración del ASIC\n\t\t\t  usb_reg5: out std_logic_vector(7 downto 0);-- DATA_byte_alto, \t\tentrada al ADCdriver\n\t\t\t  usb_reg6: out std_logic_vector(7 downto 0);-- DATA_byte_bajo, \t\tentrada al ADCdriver\n\t\t\t  usb_reg7: out std_logic_vector(7 downto 0);-- ganancia_VGA\t\t\tde configuración de la ganancia del VGA\n\t\t\t  usb_reg8: out std_logic_vector(7 downto 0);-- PulseLong_byte_alto\tpatrón del pulso de la VGA\n\t\t\t  usb_reg9: out std_logic_vector(7 downto 0);-- PulseLong_byte_bajo\n\t\t\t  usb_reg10: out std_logic_vector(7 downto 0);--Period_byte_alto\t\tperíodo de repetición del pulso de la VGA\n\t\t\t  usb_reg11: out std_logic_vector(7 downto 0);--Perido_byte_bajo\n\t\t\t  usb_reg12: out std_logic_vector(7 downto 0);--ventana_byte2\t\t\tSCALERS: ventana\n\t\t\t  usb_reg13: out std_logic_vector(7 downto 0);--ventana_byte1\t\n\t\t\t  usb_reg14: out std_logic_vector(7 downto 0);--ventana_byte0\n\t\t\t  usb_reg15: in std_logic_vector(7 downto 0);-- output_vector_byte_alto\tByte 1 de palabra de lectura que sale del ASIC\n\t\t\t  usb_reg16: in std_logic_vector(7 downto 0);-- output_vector_byte_bajo\tByte 0 de palabra de lectura que sale del ASIC\n\t\t\t  usb_reg17: in std_logic_vector(7 downto 0);-- output0_byte_alto\t\tSCALERS: salidas\n\t\t\t  usb_reg18: in std_logic_vector(7 downto 0);-- output0_byte_bajo\n\t\t\t  usb_reg19: in std_logic_vector(7 downto 0);-- output1_byte_alto\n\t\t\t  usb_reg20: in std_logic_vector(7 downto 0);-- output1_alto_bajo \n\t\t\t  usb_reg21: in std_logic_vector(7 downto 0);-- output2_byte_alto \n\t\t\t  usb_reg22: in std_logic_vector(7 downto 0);-- output2_alto_bajo \n\t\t\t  usb_reg23: in std_logic_vector(7 downto 0);-- para el canal_0 del ADCdriver\n\t\t\t  usb_reg24: in std_logic_vector(7 downto 0);\n\t\t\t  usb_reg25: in std_logic_vector(7 downto 0);-- para el canal_1 del ADCdriver\n\t\t\t  usb_reg26: in std_logic_vector(7 downto 0);\n\t\t\t  usb_reg27: in std_logic_vector(7 downto 0);-- para el canal_2 del ADCdriver\n\t\t\t  usb_reg28: in std_logic_vector(7 downto 0);\n\t\t\t  usb_reg29: in std_logic_vector(7 downto 0);-- para el canal_3 del ADCdriver\n\t\t\t  usb_reg30: in std_logic_vector(7 downto 0);\n\t\t\t  usb_reg31: in std_logic_vector(7 downto 0);-- para el canal_4 del ADCdriver\n\t\t\t  usb_reg32: in std_logic_vector(7 downto 0);\n\t\t\t  usb_reg33: in std_logic_vector(7 downto 0);-- para el canal_5 del ADCdriver\n\t\t\t  usb_reg34: in std_logic_vector(7 downto 0);\n\t\t\t  usb_reg35: in std_logic_vector(7 downto 0);-- para el canal_6 del ADCdriver\n\t\t\t  usb_reg36: in std_logic_vector(7 downto 0);\n\t\t\t  usb_reg37: in std_logic_vector(7 downto 0);-- para el canal_7 del ADCdriver\n\t\t\t  usb_reg38: in std_logic_vector(7 downto 0);\n\t\t\t  usb_reg39: in std_logic_vector(7 downto 0);-- para el canal_8 del ADCdriver\n\t\t\t  usb_reg40: in std_logic_vector(7 downto 0);\n\t\t\t  usb_reg41: in std_logic_vector(7 downto 0);-- para el canal_9 del ADCdriver\n\t\t\t  usb_reg42: in std_logic_vector(7 downto 0);\n\t\t\t  usb_reg43: in std_logic_vector(7 downto 0);-- para el canal_10 del ADCdriver\n\t\t\t  usb_reg44: in std_logic_vector(7 downto 0)--;  \n\n     usb_reg55 => LVDSByte"
  n1 = call "TEST.TEMPERATURA.vi"("error IN"="Error IN", "input cluster"="Config Test IN") -> ("error out"=w3:errorcluster, "Temperatura"=w1:dbl, "OUT cluster 2"=w4:T1)  [unwired: 7 in]
  n2 = Unbundle By Name(w4) -> ("Config HW.Espera acceso FT"=w12:u32, "Config HW.FT_Handle"=w18:u32)
  n3 = Unbundle By Name(w4) -> ("Config Test"=w26:T4, "Execucion Test.Vasic Actual"=w25:i32)
  n4 = control-ref of="Tab Control"() -> (w19:refnum<vi>)
  n5 = Index Array(array=w26, index=w25) -> (element=w29:T5)
  n6 = control-ref of="This VI"() -> (w20:refnum<vi>)
  n7 = for "Intentos" {
    N: 3 -> [_]
    tunnel: [w61] -> w39
    tunnel: [w73] -> w37
    tunnel: [w72] -> w36
    tunnel: [w71] -> w33
    tunnel: [w70] -> w32
    tunnel: w29 -> [w69]
    tunnel: [w68] -> w24
    tunnel: w12 -> [w49]
    tunnel: [w49] -> w10
    tunnel: w18 -> [w67]
    tunnel: [w65] -> w13
    tunnel: w3 -> [w66]
    tunnel: [w64] -> w11
    stop <- w62 stop-if-true
    w58 = u16 12800  # Registro Averaging (0x3200)
    w59 = u16 26624  # Registro Setup (0x6800)
    w60 = TRUE  # Reset (T=reset)
    w82 = u16[] [5461, 9557, 13653, 17749, 21845, 25941]  # Seleccion DAC_MUX
    w83 = u16[] [65535, 65535, 65535, 32767, 63]  # Max DAC
    n8 = call "ASIC_reset inicial.vi"("Espera acceso USB"=w49, "error in"=w66, "ftHandle_in"=w67) -> ("error out"=w53:errorcluster, "ftHandle_out"=w50:u32)  [unwired: 7 in]
    n9 = Unbundle By Name(w69) -> ("IBIAS"=w55:bool, "VALUE IBIAS"=w54:u8, "Limits Max PN Min NP.Max P Upper"=w79:dbl, "Limits Max PN Min NP.Max P Lower"=w78:dbl, "Limits Max PN Min NP.Min N Upper"=w77:dbl, "Limits Max PN Min NP.Min N Lower"=w76:dbl)
    n10 = call "ASIC_CONFIGURAR IABIAS.vi"("Espera acceso USB"=w49, "error in"=w53, "IBIAS VALUE"=w54, "IBIAS"=w55, "ftHandle_in"=w50) -> ("error out"=w52:errorcluster, "ftHandle_out"=w51:u32)  [unwired: 5 in]
    n11 = call "ADC_inicialización Setup-Averaging.vi"("ftHandle_in 2"=w51, "Espera acceso USB"=w49, "Reset (T=reset)"=w60, "Registro Setup (0x6800)"=w59, "Registro Averaging (0x3200)"=w58, "error in 2"=w52) -> ("ftHandle_out"=w57:u32, "error out"=w56:errorcluster)  [unwired: 8 in]
    n12 = for {
      tunnel: w83 -> [w119] mode=indexing
      tunnel: w49 -> [w113]
      tunnel: w57 -> [w111]
      tunnel: [w110] -> w80
      tunnel: w56 -> [w118]
      tunnel: [w117] -> w81
      i -> [w116]
      stop <- w109 stop-if-true
      n13 = To Unsigned Byte Integer(number=w116) -> (unsigned 8bit integer=w115:u8)
      n14 = Split Number(x=w119) -> (hi(x)=w120:u8, lo(x)=w121:u8)
      n15 = Add(x=w115, y=u8 97 ("devNum_in")) -> (x+y=w112:u8)
      n16 = global read "Global.Salir Ya.vi" "Cancel"() -> (w109:bool)
      n17 = call "ASIC_WRITE_CHECK.vi"("ftHandle_in"=w111, "Direccion Registro Asic"=w112, "Byte Alto"=w120, "Byte Bajo"=w121, "error in"=w118, "Espera acceso USB 2"=w113) -> ("ftHandle_out"=w110:u32, "error out"=w117:errorcluster)  [unwired: 11 in, 1 out]
    }
    n18 = for {
      tunnel: w82 -> [w106] mode=indexing
      tunnel: w49 -> [w101]
      tunnel: [w94] -> w73 mode=indexing
      tunnel: [w93] -> w72 mode=indexing
      tunnel: [w89] -> w68 mode=indexing
      tunnel: w80 -> [w104]
      tunnel: [w97] -> w65
      tunnel: w81 -> [w105]
      tunnel: [w96] -> w64
      i -> [w92]
      stop <- w84 stop-if-true
      n19 = Split Number(x=w106) -> (hi(x)=w107:u8, lo(x)=w108:u8)
      n20 = call "ASIC_WRITE_CHECK.vi"("ftHandle_in"=w104, "Direccion Registro Asic"=u8 96 ("devNum_in"), "Byte Alto"=w107, "Byte Bajo"=w108, "error in"=w105, "Espera acceso USB 2"=w101) -> ("ftHandle_out"=w102:u32, "error out"=w103:errorcluster)  [unwired: 11 in, 1 out]
      n21 = To Unsigned Byte Integer(number=w92) -> (unsigned 8bit integer=w88:u8)
      n22 = call "ADC_Conversion y leer.vi"("ftHandle_in 2"=w102, "Espera acceso USB"=w101, "Registro Conversion (0xD000)"=u16 53248, "error in 2"=w103) -> ("ftHandle_out"=w97:u32, "Datos Canal (V)"=w100:dbl[], "error out"=w96:errorcluster)  [unwired: 6 in, 3 out]
      n23 = Increment(x=w88) -> (x+1=w85:u8)
      n24 = Multiply(x=w85, y=8.3) -> (x*y=w86:dbl)
      n25 = global read "Global.Salir Ya.vi" "Cancel"() -> (w84:bool)
      n26 = Index Array(array=w100, index #1=4 ("index"), index #2=5 ("index")) -> (element #1=w94:dbl, element #2=w93:dbl)
      n27 = local write "Progress barr"(w86) -> ()
      n28 = local write "Progress %"(w86) -> ()
      n29 = Bundle By Name(cluster=cluster{"DAC THx":u8} {"DAC THx"=0}, "DAC THx"=w88) -> (w89:cluster{"DAC THx":u8})
    }
    n30 = In Range and Coerce(upper limit=w79, x=w73, lower limit=w78) -> (In Range?=w71:bool[])  [unwired: 1 out]
    n31 = In Range and Coerce(upper limit=w77, x=w72, lower limit=w76) -> (In Range?=w70:bool[])  [unwired: 1 out]
    n32 = global read "Global.Salir Ya.vi" "Cancel"() -> (w63:bool)
    n33 = And Array Elements(Boolean array=w71) -> (logical AND=w74:bool)
    n34 = And Array Elements(Boolean array=w70) -> (logical AND=w75:bool)
    n35 = And(x=w74, y=w75) -> (x .and. y?=w61:bool)
    n36 = Or(x=w63, y=w61) -> (x .or. y?=w62:bool)
  }
  "Max P Min N" <- w39
  n37 = property class="VI"(reference=w20, "Front Panel.ShowMenuBar"=w23, "TB.Visible"=w23, "Front Panel.TitleBarVis"=TRUE ("Front Panel Window:Title Bar Visible"), "Front Panel.Title"="TEST ASIC. Max P Min N / Max N Min P" ("Front Panel Window:Title")) -> ()  [unwired: 1 in, 2 out]
  n38 = call "WINDOWS.AUTO SIZE.vi"("Error In"=w3, "TAB.AutoAjuste"=w19, "This VI"=w20) -> ()  [unwired: 4 in, 1 out]
  n39 = disable-structure shown="Disabled" {
    frame Disabled {
      n40 = Unbundle By Name() -> ()  [unwired: 1 in, 4 out]
      n41 = Unbundle By Name() -> ()  [unwired: 1 in, 4 out]
    }
    frame Enabled {
    }
  }
  n42 = for "Intentos" {
    N: 3 -> [_]
    tunnel: [w134] -> w38
    tunnel: [w143] -> w35
    tunnel: [w142] -> w34
    tunnel: [w141] -> w31
    tunnel: [w140] -> w30
    tunnel: w29 -> [w139]
    tunnel: w10 -> [w127]
    tunnel: [w127] -> w8
    tunnel: w13 -> [w138]
    tunnel: [w151] -> w44
    tunnel: w11 -> [w137]
    tunnel: [w150] -> w43
    stop <- w136 stop-if-true
    w131 = u16 12800  # Registro Averaging (0x3200)
    w132 = u16 26624  # Registro Setup (0x6800)
    w133 = TRUE  # Reset (T=reset)
    w153 = u16[] [6826, 10922, 15018, 19114, 23210, 27306]  # Seleccion DAC_MUX
    w155 = u16[] [0, 0, 0, 32767, 63]  # Min DAC
    # "CANAL B"
    # "CANAL A"
    n43 = Unbundle By Name(w139) -> ("IBIAS"=w123:bool, "VALUE IBIAS"=w122:u8, "Limits Max PN Min NP.Min P Upper"=w149:dbl, "Limits Max PN Min NP.Max N Lower"=w148:dbl, "Limits Max PN Min NP.Max N Upper"=w147:dbl, "Limits Max PN Min NP.Max N Lower"=w146:dbl)
    n44 = call "ASIC_reset inicial.vi"("Espera acceso USB"=w127, "error in"=w137, "ftHandle_in"=w138) -> ("error out"=w124:errorcluster, "ftHandle_out"=w128:u32)  [unwired: 7 in]
    n45 = call "ASIC_CONFIGURAR IABIAS.vi"("Espera acceso USB"=w127, "error in"=w124, "IBIAS VALUE"=w122, "IBIAS"=w123, "ftHandle_in"=w128) -> ("error out"=w125:errorcluster, "ftHandle_out"=w126:u32)  [unwired: 5 in]
    n46 = call "ADC_inicialización Setup-Averaging.vi"("ftHandle_in 2"=w126, "Espera acceso USB"=w127, "Reset (T=reset)"=w133, "Registro Setup (0x6800)"=w132, "Registro Averaging (0x3200)"=w131, "error in 2"=w125) -> ("ftHandle_out"=w130:u32, "error out"=w129:errorcluster)  [unwired: 8 in]
    n47 = for {
      tunnel: w155 -> [w190] mode=indexing
      tunnel: w127 -> [w184]
      tunnel: w129 -> [w189]
      tunnel: [w188] -> w152
      tunnel: w130 -> [w182]
      tunnel: [w181] -> w154
      i -> [w187]
      stop <- w180 stop-if-true
      n48 = To Unsigned Byte Integer(number=w187) -> (unsigned 8bit integer=w186:u8)
      n49 = Split Number(x=w190) -> (hi(x)=w191:u8, lo(x)=w192:u8)
      n50 = Add(x=w186, y=u8 97 ("devNum_in")) -> (x+y=w183:u8)
      n51 = global read "Global.Salir Ya.vi" "Cancel"() -> (w180:bool)
      n52 = call "ASIC_WRITE_CHECK.vi"("ftHandle_in"=w182, "Direccion Registro Asic"=w183, "Byte Alto"=w191, "Byte Bajo"=w192, "error in"=w189, "Espera acceso USB 2"=w184) -> ("ftHandle_out"=w181:u32, "error out"=w188:errorcluster)  [unwired: 11 in, 1 out]
    }
    n53 = for {
      tunnel: w153 -> [w177] mode=indexing
      tunnel: w127 -> [w172]
      tunnel: [w164] -> w143 mode=indexing
      tunnel: [w163] -> w142 mode=indexing
      tunnel: w154 -> [w175]
      tunnel: [w167] -> w151
      tunnel: w152 -> [w176]
      tunnel: [w166] -> w150
      i -> [w160]
      stop <- w156 stop-if-true
      n54 = Split Number(x=w177) -> (hi(x)=w178:u8, lo(x)=w179:u8)
      n55 = call "ASIC_WRITE_CHECK.vi"("ftHandle_in"=w175, "Direccion Registro Asic"=u8 96 ("devNum_in"), "Byte Alto"=w178, "Byte Bajo"=w179, "error in"=w176, "Espera acceso USB 2"=w172) -> ("ftHandle_out"=w173:u32, "error out"=w174:errorcluster)  [unwired: 11 in, 1 out]
      n56 = Increment(x=w160) -> (x+1=w162:i32)
      n57 = Multiply(x=w162, y=8.3) -> (x*y=w159:dbl)
      n58 = call "ADC_Conversion y leer.vi"("ftHandle_in 2"=w173, "Espera acceso USB"=w172, "Registro Conversion (0xD000)"=u16 53248, "error in 2"=w174) -> ("ftHandle_out"=w167:u32, "Datos Canal (V)"=w170:dbl[], "error out"=w166:errorcluster)  [unwired: 6 in, 3 out]
      n59 = Add(x=w159, y=50.0) -> (x+y=w157:dbl)
      n60 = global read "Global.Salir Ya.vi" "Cancel"() -> (w156:bool)
      n61 = Index Array(array=w170, index #1=4 ("index"), index #2=5 ("index")) -> (element #1=w164:dbl, element #2=w163:dbl)
      n62 = local write "Progress barr"(w157) -> ()
      n63 = local write "Progress %"(w157) -> ()
    }
    n64 = In Range and Coerce(upper limit=w149, x=w143, lower limit=w148) -> (In Range?=w141:bool[])  [unwired: 1 out]
    n65 = In Range and Coerce(upper limit=w147, x=w142, lower limit=w146) -> (In Range?=w140:bool[])  [unwired: 1 out]
    n66 = And Array Elements(Boolean array=w140) -> (logical AND=w145:bool)
    n67 = global read "Global.Salir Ya.vi" "Cancel"() -> (w135:bool)
    n68 = And Array Elements(Boolean array=w141) -> (logical AND=w144:bool)
    n69 = And(x=w144, y=w145) -> (x .and. y?=w134:bool)
    n70 = Or(x=w135, y=w134) -> (x .or. y?=w136:bool)
  }
  "Min P Max N" <- w38
  n71 = Unbundle By Name(w4) -> ("Result"=w27:T6, "Execucion Test.Vasic Actual"=w42:i32)
  n72 = Split Number(x=u16 1855 ("devNum_in")) -> (hi(x)=w48:u8, lo(x)=w47:u8)
  n73 = call "ASIC_WRITE_CHECK.vi"("ftHandle_in"=w44, "Direccion Registro Asic"=u8 101 ("devNum_in"), "Byte Alto"=w48, "Byte Bajo"=w47, "error in"=w43, "Espera acceso USB 2"=w8) -> ("ftHandle_out"=w17:u32, "error out"=w16:errorcluster)  [unwired: 11 in, 1 out]
  n74 = call "ASIC_reset inicial.vi"("Espera acceso USB"=w8, "error in"=w16, "ftHandle_in"=w17) -> ("error out"=→"Error OUT":errorcluster, "ftHandle_out"=w14:u32)  [unwired: 7 in]
  n75 = Index Array(array=w27, index=w42) -> (element=w41:T7)
  n76 = Bundle By Name(cluster=w41, "Test Max-Min PN.Max P Mini N OK"=w39, "Test Max-Min PN.Min P Max N OK"=w38, "Test Max-Min PN.PTHT Max P Min N"=w37, "Test Max-Min PN.PTHT Max P Min N OK"=w33, "Test Max-Min PN.NTHT Max P Min N"=w36, "Test Max-Min PN.NTHT Max P Min N OK"=w32, "Test Max-Min PN.PTHT Max N Min P"=w35, "Test Max-Min PN.PTHT Max N Min P OK"=w31, "Test Max-Min PN.NTHT Max N Min P"=w34, "Test Max-Min PN.NTHT Max N Min P OK"=w30, "Test Max-Min PN.Ref"=w24, "info temp.T Asic Max Min N P"=w1) -> (w40:T7)
  n77 = Insert Into Array(array=w27, index=w42, new element=w40) -> (w28:T6)
  n78 = Bundle By Name(cluster=w4, "Result"=w28, "Config HW.FT_Handle"=w14) -> (w6:T1)
  "Config Test OUT" <- w6
  n79 = flat-sequence {
    tunnel: w6 -> [_]
    frame #0 {
      n80 = control-ref of="This VI"() -> (w193:refnum<vi>)
      n81 = invoke class="VI" method="FP.Close"(reference=w193) -> ()  [unwired: 2 in, 3 out]
    }
  }
